vi "Load VI State.vi"(8 "error in (no error)":errorcluster, 10 "state file path (<application path>\\<vi name>.state)":path, 11 "vi reference (caller VI)":refnum<vi>) -> (0 "error out":errorcluster)   [LabVIEW 2015, in "PL Utility.lvlib"]
doc: "Loads control and indicator values from binary file specified by <b>state file path</b> for the VI specified by <b>vi reference</b>."
uses:
  PL Utility.lvlib
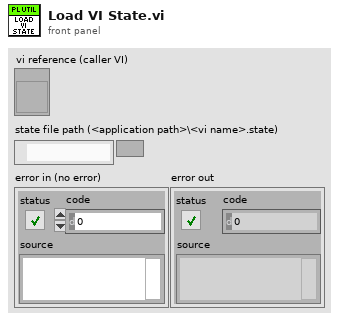
[diagram p1: front panel]
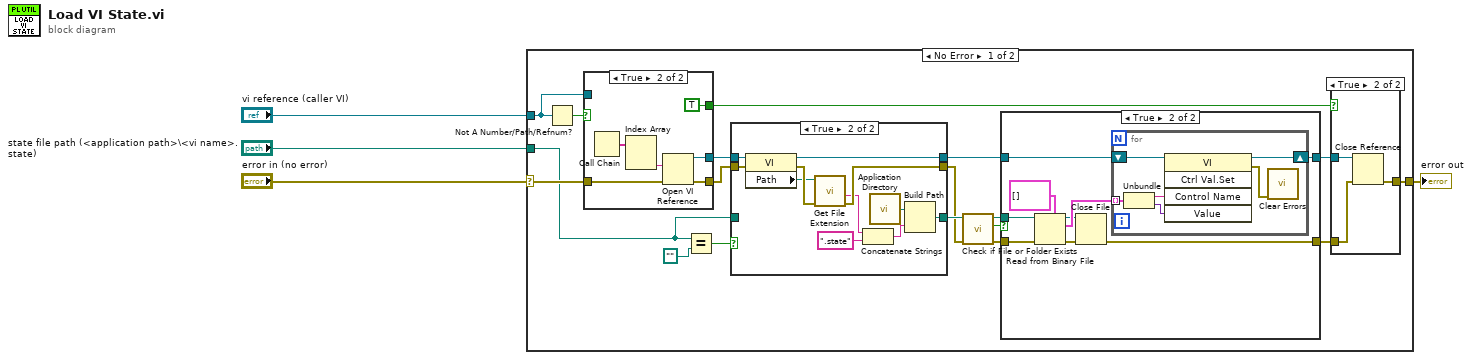
[diagram p0: block diagram]
diagram:
  n1 = case shown="No Error" "error in (no error)" {
    selector: "error in (no error)" -> [w20 w66]
    tunnel: [w13 w66] -> w3
    tunnel: "state file path (<application path>\\<vi name>.state)" -> [w15 _]
    tunnel: "vi reference (caller VI)" -> [w21 _]
    frame No Error {
      n2 = Not A Number/Path/Refnum?(number/path/refnum=w21) -> (NaN/Path/Refnum?=w22:bool)
      n3 = case shown="True" w22 {
        tunnel: w21 -> [w59 _]
        tunnel: [w59 w63] -> w19
        tunnel: w20 -> [w58 w62]
        tunnel: [w58 w61] -> w18
        tunnel: [_ TRUE] -> w14
        frame False {
        }
        frame True {
          n4 = Call Chain() -> (call chain=w65:string[])
          n5 = Index Array(array=w65) -> (element #2=w64:string)  [unwired: 2 in, 1 out]
          n6 = Open VI Reference(vi path=w64, error in (no error)=w62) -> (vi reference=w63:refnum<vi>, error out=w61:errorcluster)  [unwired: 4 in]
        }
      }
      n7 = Equal?(x=w15, y=path "") -> (x = y?=w16:bool)
      n8 = case shown="True" w16 {
        tunnel: w19 -> [w45 w57]
        tunnel: w18 -> [w44 w56]
        tunnel: w15 -> [w46 _]
        tunnel: [w46 w53] -> w12
        tunnel: [w45 w55] -> w6
        tunnel: [w44 w50] -> w11
        frame False {
        }
        frame True {
          n9 = property class="VI"(reference=w57, error in=w56) -> (reference out=w55:refnum<vi>, error out=w52:errorcluster, "Path"=w51:path)
          n10 = call <vilib>:"Get File Extension.vi"("error in (no error)"=w52, "file"=w51) -> ("error out"=w50:errorcluster, "filename without extension"=w48:string)  [unwired: 5 in, 3 out]
          n11 = Concatenate Strings(w48, ".state" ("string")) -> (w49:string)
          n12 = call <vilib>:"Application Directory.vi"() -> ("Application Directory"=w54:path)
          n13 = Build Path(base path=w54, name or relative path=w49) -> (appended path=w53:path)
        }
      }
      n14 = call <vilib>:"Check if File or Folder Exists.vi"("error in (no error)"=w11, "path"=w12) -> ("error out"=w8:errorcluster, "file or folder exists?"=w10:bool, "dup path"=w9:path)  [unwired: 7 in]
      n15 = case shown="True" w10 {
        tunnel: w9 -> [_ w32]
        tunnel: w8 -> [w24 w31]
        tunnel: [w24 w25] -> w7
        tunnel: w6 -> [w23 w30]
        tunnel: [w23 w28] -> w5
        frame False {
        }
        frame True {
          n16 = Read from Binary File(5:cluster{"Name":string, "Variant Data":variant}[] [] ("appended array"), 8:w31, 11:w32) -> (0:w26:errorcluster, 2:w29:cluster{"Name":string, "Variant Data":variant}[], 3:w27:refnum<file>)  [unwired: 3 in, 1 out]
          n17 = Close File(refnum=w27, error in=w26) -> (error out=w25:errorcluster)  [unwired: 1 out]
          n18 = for {
            shift-right: [w38] -> w28
            shift-left: w30 -> [w39]
            tunnel: w29 -> [w36] mode=indexing
            n19 = Unbundle(w36) -> ("Name"=w35:string, "Variant Data"=w34:variant)
            n20 = invoke class="VI" method="Ctrl Val.Set"(reference=w39, "Control Name"=w35, "Value"=w34) -> (reference out=w38:refnum<vi>, error out=w37:errorcluster)  [unwired: 2 in, 3 out]
            n21 = call <vilib>:"Clear Errors.vi"("error in (no error)"=w37) -> ()  [unwired: 5 in, 2 out]
          }
        }
      }
      n22 = case shown="True" w14 {
        tunnel: w7 -> [w40 w41]
        tunnel: [w40 w42] -> w13
        tunnel: w5 -> [_ w43]
        frame False {
        }
        frame True {
          n23 = Close Reference(reference=w43, error in (no error)=w41) -> (error out=w42:errorcluster)
        }
      }
    }
    frame Error {
    }
  }
  "error out" <- w3
